vi "Left Tilt Motor Tester.vi"() -> ()   [LabVIEW 2015]
uses:
  <vilib>/Platform/TimedLoop/XDataNode/timing_clust.ctl
  <vilib>/Platform/TimedLoop/XDataNode/nitl_modes.ctl
  <vilib>/Platform/TimedLoop/XDataNode/wakeup.ctl
  <vilib>/Utility/error.llb/Error Cluster From Error Code.vi
  <vilib>/myRIO/Common/Instrument Driver Framework/myRIO v1.0/DIO/vis/myRIO v1.0 Write DIO.vi
  <vilib>/platform/TimedLoop/XDataNode/XDataNode.xnode
  <vilib>/myRIO/Instrument Drivers/Onboard IO/DIO/DIO.lvlib
  <vilib>/Platform/TimedLoop/XDataNode/XDNodeRunTimeDep.lvlib
panel:
  in  "STOP":bool
  in  "Direction\n(Toggle)":bool
  in  "Pulse Width\n(uSec)":u16(slide)=50 scale=500.0..2000.0
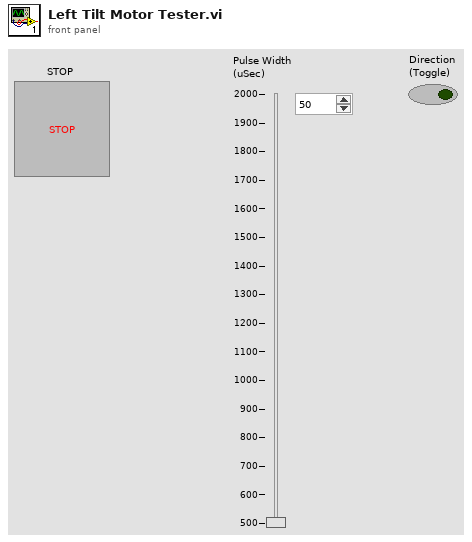
[diagram p1: front panel]
types:
  T1 = typedef "DIO.lvlib/DIO Reference.ctl" = cluster{"myRIO Reference":T2, "DIO Channels List":T6}
  T2 = typedef "myRIO Generic Hardware Reference.ctl" = cluster{"myRIO Model":T3, "myRIO Hardware Reference":T4}
  T3 = typedef "Hardware Version Enum.ctl" = enum16{"Unknown", "myRIO-1900", "myRIO-1950", "roboRIO"}
  T4 = typedef "myRIO v1.0 Reference.ctl" = cluster{"Generic FPGA Reference":T5, "Allow multiple opens":bool}
  T5 = typedef "Generic FPGA Reference.ctl" = refnum<k20>
  T6 = typedef "DIO Channels List.ctl" = T7[]
  T7 = typedef "DIO Channels Enum.ctl" = enum16{"Not Connected", "C/DIO0", "C/DIO1", "C/DIO2", "C/DIO3", "C/DIO4", "C/DIO5", "C/DIO6", "C/DIO7", "A/DIO0", "A/DIO1", "A/DIO2", "A/DIO3", "A/DIO4", "A/DIO5", "A/DIO6", "A/DIO7", "A/DIO8", "A/DIO9", "A/DIO10", "A/DIO11", "A/DIO12", "A/DIO13", "A/DIO14", "A/DIO15", "B/DIO0", "B/DIO1", "B/DIO2", "B/DIO3", "B/DIO4", "B/DIO5", "B/DIO6", "B/DIO7", "B/DIO8", "B/DIO9", "B/DIO10", "B/DIO11", "B/DIO12", "B/DIO13", "B/DIO14", "B/DIO15", "LED0", "LED1", "LED2", "LED3", "Button0", "DIO/DIO0", "DIO/DIO1", "DIO/DIO2", "DIO/DIO3", "DIO/DIO4", "DIO/DIO5", "DIO/DIO6", "DIO/DIO7", "DIO/DIO8", "DIO/DIO9", "SPI/CS0", "SPI/CS1", "SPI/CS2", "SPI/CS3", "LED RADIO (Green)", "LED RADIO (Red)", "LED COMM (Green)", "LED COMM (Red)", "LED MODE (Green)", "LED MODE (Red)"}
  T8 = typedef "XDNodeRunTimeDep.lvlib/timing_clust.ctl" = cluster{"Expected End [f-1]":u64, "Actual End [f-1]":u64, "Finished Late? [f-1]":bool, "Expected End [i-1]":u64, "Actual End [i-1]":u64, "Finished Late? [i-1]":bool, "Expected Start [i]":u64, "Actual Start [i]":u64, "Expected Start [f]":u64, "Actual Start [f]":u64, "Source Name":string, "Structure Name":string, "Period":i64, "Deadline":i64, "Offset":i64, "Start":i64, "Priority":i32, "Timeout":i32, "Mode":T9, "Wakeup Reason":T10, "Error":errorcluster, "Source Type":string, "Secondary Source Type":string, "Global End Time":u64, "Global Start Time":u64, "Frame Duration":u64, "Iteration Duration":u64, "Assigned CPU":i32, "I/O Scan Engine Mode":u32}
  T9 = typedef "XDNodeRunTimeDep.lvlib/nitl_modes.ctl" = enum32{"No Change", "Process missed periods, maintain original phase", "Discard missed periods, maintain original phase", "Process missed periods, ignore original phase", "Discard missed periods, ignore original phase"}
  T10 = typedef "XDNodeRunTimeDep.lvlib/wakeup.ctl" = enum32{"Normal", "Aborted", "Asynchronous wakeup", "Timing source error", "Timed loop error", "Timeout"}
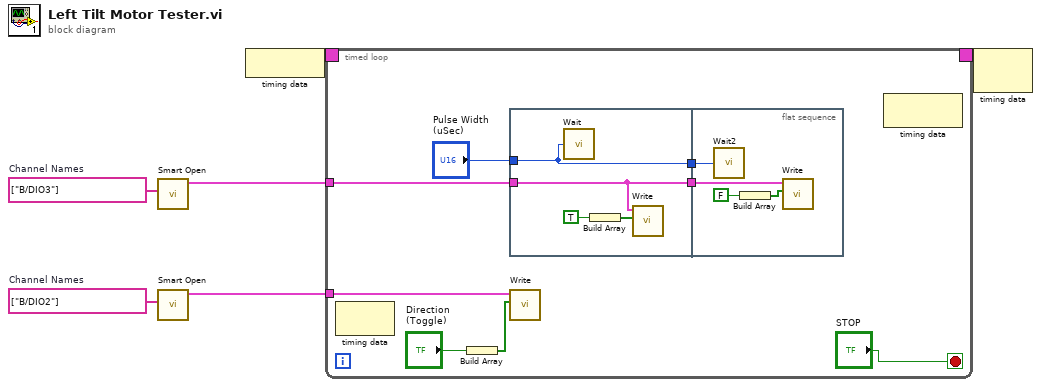
[diagram p0: block diagram]
diagram:
  w2 = tag[] ["B/DIO2"]  # Channel Names
  w4 = tag[] ["B/DIO3"]  # Channel Names
  n1 = call <vilib>:"Smart Open.vi"("Channel Names"=w4) -> ("DIO Ref Out"=w3:T1)  [unwired: 9 in, 1 out]
  n2 = call <vilib>:"Smart Open.vi"("Channel Names"=w2) -> ("DIO Ref Out"=w1:T1)  [unwired: 9 in, 1 out]
  n3 = node-c288() -> (w6:T8)
  n4 = timed-loop {
    timing: w6 -> [_]
    timing-out: [_] -> w5
    tunnel: w3 -> [w11]
    tunnel: w1 -> [w7]
    stop <- "STOP" stop-if-true
    n5 = node-c288() -> ()  [unwired: 1 in, 1 out]
    n6 = Build Array("Direction\n(Toggle)") -> (w8:bool[])
    n7 = flat-sequence {
      tunnel: [w20] -> w14
      tunnel: "Pulse Width\n(uSec)" -> [w20]
      tunnel: w11 -> [w17]
      tunnel: [w17] -> w10
      tunnel: w14 -> [w24]
      tunnel: w10 -> [w21]
      frame #0 {
        n8 = call "Wait"("Count(uSec)"=w20) -> ()  [unwired: 1 out]
        n9 = Build Array(TRUE ("A/DIO1 (Pin 13)")) -> (w18:bool[])
        n10 = call <vilib>:"Write.vi"("Values"=w18, "DIO Ref In"=w17) -> ()  [unwired: 7 in, 2 out]
      }
      frame #1 {
        n11 = call "Wait2"("Count(uSec)"=w24) -> ()  [unwired: 1 out]
        n12 = Build Array(FALSE ("A/DIO2 (Pin 15)")) -> (w22:bool[])
        n13 = call <vilib>:"Write.vi"("Values"=w22, "DIO Ref In"=w21) -> ()  [unwired: 7 in, 2 out]
      }
    }
    n14 = call <vilib>:"Write.vi"("Values"=w8, "DIO Ref In"=w7) -> ()  [unwired: 7 in, 2 out]
    n15 = node-c288() -> ()  [unwired: 1 in, 1 out]
  }
  n16 = node-c288(w5) -> ()  [unwired: 1 out]
